vi "Configure Measurement Statistics.vi"(8 "error in (no error)":errorcluster, 9 "Enable Relative Standard Deviation (F: Disable)":bool, 10 "Statistics Count (Inf)":dbl=inf, 11 "VISA resource name":refnum<visa-resource-name>) -> (0 "error out":errorcluster, 3 "VISA resource name out":refnum<visa-resource-name>)   [LabVIEW 2015, in "Agilent 2000 3000 X-Series.lvlib"]
doc: "Configure the measurement statistics settings.\n\nNote:\nThis VI is not supported by 1000 X Series"
uses:
  Agilent 2000 3000 X-Series.lvlib
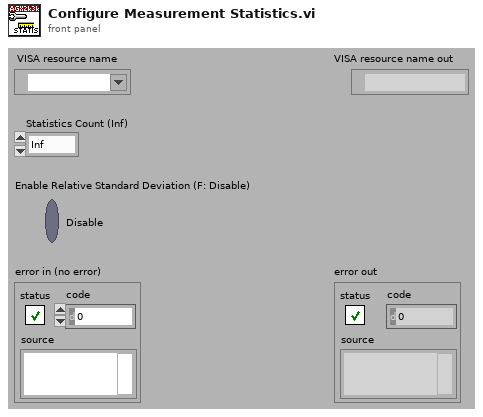
[diagram p1: front panel]
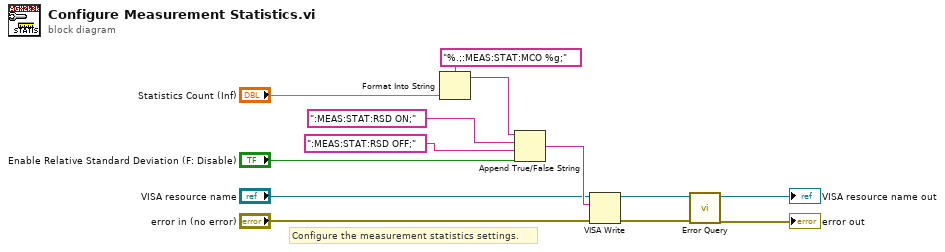
[diagram p0: block diagram]
diagram:
  # "Configure the measurement statistics settings."
  n1 = Format Into String(format string="%.;:MEAS:STAT:MCO %g;", "Statistics Count (Inf)") -> (resulting string=w11:string)  [unwired: 2 in, 1 out]
  n2 = Append True/False String(1:"Enable Relative Standard Deviation (F: Disable)", 2:":MEAS:STAT:RSD OFF;", 3:":MEAS:STAT:RSD ON;", 4:w11) -> (0:w7:string)
  n3 = VISA Write(VISA resource name="VISA resource name", write buffer=w7, error in (no error)="error in (no error)") -> (VISA resource name out=w4:refnum<visa-resource-name>, error out=w3:errorcluster)  [unwired: 1 out]
  n4 = call "Error Query.vi"("error in (no error)"=w3, "VISA resource name"=w4) -> ("error out"=→"error out":errorcluster, "VISA resource name out"=→"VISA resource name out":refnum<visa-resource-name>)  [unwired: 8 out]
